vi "LoadParam.vi"(8 "error in (no error)":errorcluster, 10 "File Path Control":path=path "D:/USERS/MONTRI/BABYDOL/LABVIEW/EXEMPLE_ARCHITECTURE/CONFIG/config.ini", 11 "HAMAMATSU_DCAMAPI in":refnum<class "HAMAMATSU_DCAMAPI.lvclass">=refnum) -> (0 "error out":errorcluster, 3 "HAMAMATSU_DCAMAPI out":refnum<class "HAMAMATSU_DCAMAPI.lvclass">)   [LabVIEW 2020, in "HAMAMATSU_DCAMAPI.lvclass"]
uses:
  HAMAMATSU_DCAMAPI.lvclass
  HAMAMATSU_DCAMAPI.lvclass/HAMAMATSU_DCAMAPI.ctl
panel:
  in  "Scan Mode":dbl=3.0 format="%#_13g"
  out "SMD":dbl=3.0
  out "EXP 2":dbl=0.00010305882352941175
  in  "Exposure":dbl=1e-05 format="%#_13g"
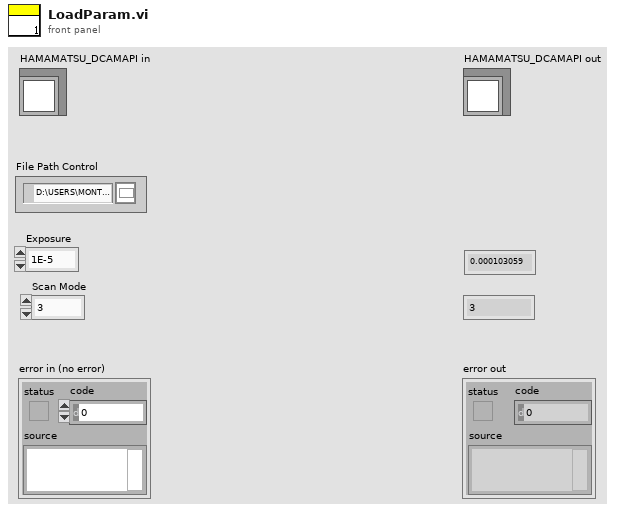
[diagram p1: front panel]
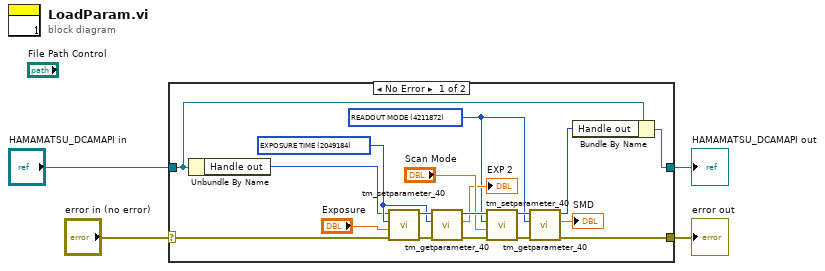
[diagram p0: block diagram]
diagram:
  n1 = case shown="No Error" "error in (no error)" {
    selector: "error in (no error)" -> [w5 w23]
    tunnel: [w8 w23] -> w3
    tunnel: "HAMAMATSU_DCAMAPI in" -> [w21 w24]
    tunnel: [w22 w24] -> w1
    frame No Error {
      w10 = u32 4211872 items=["SENSOR MODE"=4212128, "CCD MODE"=4212384, "READOUT MODE"=4211872, "ACTIVE VIEW INDEX"=4343136, "BITS PER CHANNEL"=4342976, "IMAGE PIXEL TYPE"=4343296, "BINNING"=4215968, "EXPOSURE TIME"=2049184, "CONTRAST GAIN"=3163312, "CONTRAST OFFSET"=3163328, "LIGHT MODE"=2114720, "SENSITIVITY"=2114992, "PHOTON IMAGING MODE"=2115200, "HIGH DYNAMIC RANGE MODE"=3163360, "WHITE BALANCE"=3163568, "TEMPERATURE"=2115232, "TEMPERATURE TARGET"=2115264, "SENSOR COOLER FAN"=2115296, "LINEBUNDLE HEIGHT"=4212192, "MECHANICAL SHUTTER"=2115488, "BACK FOCUS POSITION"=8422304, "TRIGGER CONNECTOR"=1066432, "TRIGGER SOURCE"=1066144, "OUTPUT TRIGGER SOURCE"=1852576, "TRIGGER GLOBAL EXPOSURE"=2049680, "FIRST TRIGGER BEHAVIOR"=2049696, "CHANNEL SYNC"=1852352, "READOUT DIRECTION"=4211904, "PRE HSYNC COUNT"=1852704] ("Parameter")
      w9 = u32 2049184 items=["SENSOR MODE"=4212128, "CCD MODE"=4212384, "READOUT MODE"=4211872, "ACTIVE VIEW INDEX"=4343136, "BITS PER CHANNEL"=4342976, "IMAGE PIXEL TYPE"=4343296, "BINNING"=4215968, "EXPOSURE TIME"=2049184, "CONTRAST GAIN"=3163312, "CONTRAST OFFSET"=3163328, "LIGHT MODE"=2114720, "SENSITIVITY"=2114992, "PHOTON IMAGING MODE"=2115200, "HIGH DYNAMIC RANGE MODE"=3163360, "WHITE BALANCE"=3163568, "TEMPERATURE"=2115232, "TEMPERATURE TARGET"=2115264, "SENSOR COOLER FAN"=2115296, "LINEBUNDLE HEIGHT"=4212192, "MECHANICAL SHUTTER"=2115488, "BACK FOCUS POSITION"=8422304, "TRIGGER CONNECTOR"=1066432, "TRIGGER SOURCE"=1066144, "OUTPUT TRIGGER SOURCE"=1852576, "TRIGGER GLOBAL EXPOSURE"=2049680, "FIRST TRIGGER BEHAVIOR"=2049696, "CHANNEL SYNC"=1852352, "READOUT DIRECTION"=4211904, "PRE HSYNC COUNT"=1852704] ("Parameter")
      n2 = Unbundle By Name(w21) -> ("Handle out"=w6:u32)
      n3 = call <userlib>:"tm_setparameter_40.vi"("error in (no error)"=w5, "Value in"="Exposure", "Parameter"=w9, "Handle in"=w6) -> ("error out"=w11:errorcluster, "Handle out"=w12:u32)  [unwired: 6 in]
      n4 = call <userlib>:"tm_getparameter_40.vi"("error in (no error)"=w11, "Parameter"=w9, "Handle in"=w12) -> ("error out"=w20:errorcluster, "Value out"=→"EXP 2":dbl, "Handle out"=w19:u32)  [unwired: 6 in]
      n5 = call <userlib>:"tm_setparameter_40.vi"("error in (no error)"=w20, "Value in"="Scan Mode", "Parameter"=w10, "Handle in"=w19) -> ("error out"=w15:errorcluster, "Handle out"=w16:u32)  [unwired: 6 in]
      n6 = call <userlib>:"tm_getparameter_40.vi"("error in (no error)"=w15, "Parameter"=w10, "Handle in"=w16) -> ("error out"=w8:errorcluster, "Value out"=→"SMD":dbl, "Handle out"=w7:u32)  [unwired: 6 in]
      n7 = Bundle By Name(cluster=w21, "Handle out"=w7) -> (w22:refnum<class "HAMAMATSU_DCAMAPI.lvclass">)
    }
    frame Error {
    }
  }
  "error out" <- w3
  "HAMAMATSU_DCAMAPI out" <- w1
